vi "SVFA Extract Tone Information.vi"   [LabVIEW 2017]
doc: "Identifies a sinusoidal component in a scaled signal. A sinusoidal component is a peak in the magnitude of the complex spectrum. This VI does not maintain state, you can use this VI in a loop to process an array of channels."
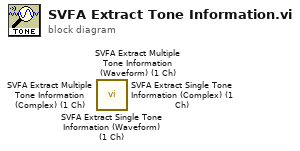
[diagram p0: block diagram]
diagram:
  n1 = call <vilib>:"SVFA Extract Single Tone Information (Waveform) (1 Ch).vi"() -> ()  [unwired: 17 in, 3 out]
  n2 = call <vilib>:"SVFA Extract Multiple Tone Information (Waveform) (1 Ch).vi"() -> ()  [unwired: 17 in, 3 out]
  n3 = call <vilib>:"SVFA Extract Multiple Tone Information (Complex) (1 Ch).vi"() -> ()  [unwired: 16 in, 4 out]
  n4 = call <vilib>:"SVFA Extract Single Tone Information (Complex) (1 Ch).vi"() -> ()  [unwired: 16 in, 4 out]
